vi "Main Controller AM.vi"(8 "Error In":errorcluster) -> (0 "Error Out":errorcluster)   [LabVIEW 2017, in "Main controller.lvlib"]
uses:
  Main controller.lvlib
  Shutter Module/Shutter.lvlib
  Monochromator/Monochromator.lvlib
  UI/UI.lvlib
  DAQ/DAQ.lvlib
  Monochromator/Controls/VISA parameters.ctl
  Serial comms/Serial comms.lvlib
  Monochromator/Controls/Grating.ctl
  Monochromator/Controls/Params.ctl
  DAQ/Controls/Params.ctl
  Scope/Scope.lvlib
  Monochromator/Controls/Type.ctl
  Scope/Controls/TPC.ctl
  Scope/Controls/Models.ctl
  Trigger/Controls/Mode.ctl
  Trigger/Trigger.lvlib
  Trigger/Controls/Params.ctl
  Scope/Controls/Params.ctl
  File IO/File IO.lvlib
  Scope/Controls/Record length.ctl
  Scope/Controls/Acquisition type.ctl
  Trigger channels.ctl
  Colour Wheel/Colour Wheel.lvlib
  Colour Wheel/Controls/Params.ctl
  Scope/Controls/Channel data.ctl
  Scope/Controls/Data.ctl
  Monochromator/Oriel/Controls/Params.ctl
  Monochromator/Oriel/Oriel (old drivers).lvlib
  Monochromator/Custom Oriel drivers/Controls/Params.ctl
  Monochromator/Custom Oriel drivers/Oriel (custom drivers).lvlib
  Monochromator/PTI/Controls/Params.ctl
  Monochromator/PTI/PTI.lvlib
  Monochromator/Controls/GratingValues.ctl
  Events/Events.lvlib
  Events/Controls/Action Refs [enum].ctl
  Test params.ctl
  CTLs/Test indicators.ctl
  Scope/Controls/Channels.ctl
  Processing/Processing.lvlib
  Colour Wheel/Controls/Colours.ctl
  Auto cycle/Controls/Steps.ctl
  Auto cycle/Auto cycle.lvlib
  Auto cycle/Controls/Checks.ctl
  C:/Project Work/icl-optical-software-rewrite/Optical Software Code Simplified/Modules/Monochromator/Cornerstone.dll
  Monochromator/Cornerstone.dll
  Shutter Module/Controls/Params.ctl
  File IO/Controls/Params.ctl
  CTLs/Params.ctl
  CTLs/Test Controls.ctl
  CTLs/Commands [enum].ctl
panel:
  out "Current step":T1
  in  "Commands":T2
  out "Standalone":bool
  out "Config out":T3={"DAQ"={"Data"={"Live"={"t0"=timestamp(0 s since 1904-01-01), "dt"=1.0, "Y"=[]}, "Accumulated"={"t0"=timestamp(0 s since 1904-01-01), "dt"=1.0, "Y"=[]}, "Averaged"={"t0"=timestamp(0 s since 1904-01-01), "dt"=1.0, "Y"=[]}, "data array"=[], "live time array"=[], "Live (decimated)"={"t0"=timestamp(0 s since 1904-01-01), "dt"=1.0, "Y"=[]}}, "Config"={"Input Config"=-1, "Card"=enum."USB-6211", "100% Reflectance Standard (V)"=1.0, "Input Channel"="Dev2/ai0", "Average number of points"=10.0, "Trigger Level (V)"=0.3, "Rate"=250000, "End Time (s)"=1.0}, "Indicators"={"Final number of points"=0.0, "Number of samples"=0.0, "dt"=0.0, "Shots"=1, "Shot counter"=0, "Test counter"=0, "Background level (V)"=0.0, "DAQ task"="", "timestamp of data"=timestamp(0 s since 1904-01-01)}}, "Shutter"={"Open command string"="", "VISA"={"Enable Termination Char (T)"=FALSE, "timeout (ms)"=0, "Resource name"="", "baud rate"=0, "data bits"=0, "parity"=0, "stop bits"=0, "flow control"=0}}, "Monochromator"={"Type"=enum."Oriel", "Wavelength (nm)"=0.0, "Grating, gr/mm"=enum."2400", "Grating mode"=enum."unknown", "Spectrum mode"={"Spectrum mode?"=FALSE, "Start wavelength (nm)"=0.0, "End wavelength (nm)"=0.0, "Wavelength step (nm)"=0.0, "Wavelength array"=[], "array index"=0}, "PTI"={"delay before read (ms)"=0, "Mono 1"={"Enable Termination Char (T)"=FALSE, "timeout (ms)"=0, "Resource name"="", "baud rate"=0, "data bits"=0, "parity"=0, "stop bits"=0, "flow control"=0}, "Mono 2"={"Enable Termination Char (T)"=FALSE, "timeout (ms)"=0, "Resource name"="", "baud rate"=0, "data bits"=0, "parity"=0, "stop bits"=0, "flow control"=0}}, "Oriel (custom)"={"reference"=refnum}, "Oriel (old)"={"configuration file path"=path ""}, "Force wavelength confirmation (PTI)?"=FALSE}, "Test"={"Config"={"Amplification Factor"=0.0, "100% reflectance standard"=0.0, "Calculation Method"=enum."Reflectance", "Option to discard new data?"=FALSE, "Mode"=enum."Spectrum", "Number of averages"=0, "B Test?"=FALSE}, "Indicators"={"DAQ Background Level (V)"=0.0, "A-Test Counter"=0, "B-test counter"=0, "Type"=enum."A-test", "Scope Background Level (Amps)"=2.0, "TAS only?"=FALSE}}, "Scope"={"Config"={"VISA resource"="USB0::0x0699::0x039D::C010764::INSTR", "Model"=enum."DPO 2012B", "Timebase"=0.0004, "Timeout (ms)"=60000, "TAS"={"Vertical Range (10.0 V)"=2.0, "Vertical Offset (0.0 divs)"=0.0, "Bandwidth"=0, "Probe Attenuation (10.0)"=1.0, "Vertical Coupling"=1, "Impedance"=0, "Multiplication factor"=1.0, "Channel"=enum."Channel 1"}, "TPC"={"Vertical Range (10.0 V)"=2.0, "Vertical Offset (0.0 divs)"=0.0, "Bandwidth"=0, "Probe Attenuation (10.0)"=1.0, "Vertical Coupling"=1, "Impedance"=0, "Multiplication factor"=1.0, "Channel"=enum."None"}, "Trigger"={"Mode"=enum."Laser (TAS)", "Source "=enum."Aux", "PIA mode"={"Test LEDs"=FALSE, "LED line"="", "LED off (s)"=0.0, "LED on (s)"=0.0}, "Threshold (V)"=0.8}}, "Indicators"={"Setup"={"Final number of points"=0.0, "Pretrigger points"=0.0, "Number of readouts"=0, "Model"={"Acquisition Type"=4, "Record length (points)"=1000, "Averages on scope"=4, "Average number of points"=10.0}}, "timestamp of data"=timestamp(0 s since 1904-01-01)}, "Data"={"TPC"={"Live data"={"t0"=timestamp(0 s since 1904-01-01), "dt"=1.0, "Y"=[]}, "Averaged data"={"t0"=timestamp(0 s since 1904-01-01), "dt"=1.0, "Y"=[]}, "Accumulated data"={"t0"=timestamp(0 s since 1904-01-01), "dt"=1.0, "Y"=[]}, "Final data"={"t0"=timestamp(0 s since 1904-01-01), "dt"=1.0, "Y"=[]}}, "TAS"={"Live data"={"t0"=timestamp(0 s since 1904-01-01), "dt"=1.0, "Y"=[]}, "Averaged data"={"t0"=timestamp(0 s since 1904-01-01), "dt"=1.0, "Y"=[]}, "Accumulated data"={"t0"=timestamp(0 s since 1904-01-01), "dt"=1.0, "Y"=[]}, "Final data"={"t0"=timestamp(0 s since 1904-01-01), "dt"=1.0, "Y"=[]}}, "Time arrays"={"Time array (decimated)"=[], "waveform"={"t0"=timestamp(0 s since 1904-01-01), "dt"=1.0, "Y"=[]}}}, "Test"={"Config"={"Amplification Factor"=0.0, "100% reflectance standard"=0.0, "Calculation Method"=enum."Reflectance", "Option to discard new data?"=FALSE, "Mode"=enum."Spectrum", "Number of averages"=100}, "Indicators"={"DAQ Background Level (V)"=2.0, "A-Test Counter"=2, "B-test counter"=2, "Type"=enum."A-test", "Scope Background Level (Amps)"=2.0, "TAS only?"=FALSE}, "Stop Measurement"=FALSE, "Stop Measurement 2"=FALSE}}, "Colour wheel"={"Reference"=0, "Wavelength Enum"=enum."435"}, "File IO"={"Output Folder"=path "C:/Users/Abigail/Documents/Imperial Optical software/Optical Software Code Simplified/Output", "Error file"=path "C:/Users/Abigail/Documents/Imperial Optical software/Optical Software Code Simplified/Error Log.txt", "Config file"=path "C:/Users/Abigail/Documents/Imperial Optical software/Optical Software Code Simplified/Config.ini", "File prefix"="", "Waveform read"={"t0"=timestamp(0 s since 1904-01-01), "dt"=1.0, "Y"=[]}}} {"Scope"."Indicators"."Setup"."Model"."Record length (points)" items=["1000"=1, "10,000"=10, "100,000"=100, "1,000,000"=1000, "5,000,000"=5000, "10,000,000"=10000]; "Scope"."Indicators"."Setup"."Model"."Acquisition Type" items=["Sample", "Peak Detect", "Hi Res", "Envelope", "Average"]; "Scope"."Config"."Trigger"."Threshold (V)" format="%#_3f"; "Scope"."Config"."TPC"."Impedance" items=["1M", "75", "50"]; "Scope"."Config"."TPC"."Vertical Coupling" items=["AC", "DC", "Ground"]; "Scope"."Config"."TPC"."Bandwidth" items=["FULL", "250 MHz", "150 MHz", "20 MHz"]; "Scope"."Config"."TAS"."Impedance" items=["1M", "75", "50"]; "Scope"."Config"."TAS"."Vertical Coupling" items=["AC", "DC", "Ground"]; "Scope"."Config"."TAS"."Bandwidth" items=["FULL", "250 MHz", "150 MHz", "20 MHz"]; "Scope"."Config"."Timebase" format="%^#_3e"; "Monochromator"."PTI"."Mono 2"."flow control" items=["None"=0, "XON/XOFF"=1, "RTS/CTS"=2, "DTR/DSR"=4]; "Monochromator"."PTI"."Mono 2"."stop bits" items=["1.0"=10, "1.5"=15, "2.0"=20]; "Monochromator"."PTI"."Mono 2"."parity" items=["None", "Odd", "Even", "Mark", "Space"]; "Monochromator"."PTI"."Mono 1"."flow control" items=["None"=0, "XON/XOFF"=1, "RTS/CTS"=2, "DTR/DSR"=4]; "Monochromator"."PTI"."Mono 1"."stop bits" items=["1.0"=10, "1.5"=15, "2.0"=20]; "Monochromator"."PTI"."Mono 1"."parity" items=["None", "Odd", "Even", "Mark", "Space"]; "Shutter"."VISA"."flow control" items=["None"=0, "XON/XOFF"=1, "RTS/CTS"=2, "DTR/DSR"=4]; "Shutter"."VISA"."stop bits" items=["1.0"=10, "1.5"=15, "2.0"=20]; "Shutter"."VISA"."parity" items=["None", "Odd", "Even", "Mark", "Space"]; "DAQ"."Config"."Input Config" items=["default"=-1, "RSE"=10083, "NRSE"=10078, "Differential"=10106, "Pseudodifferential"=12529]}
  # "#TODO: \"stop[current-test]\""
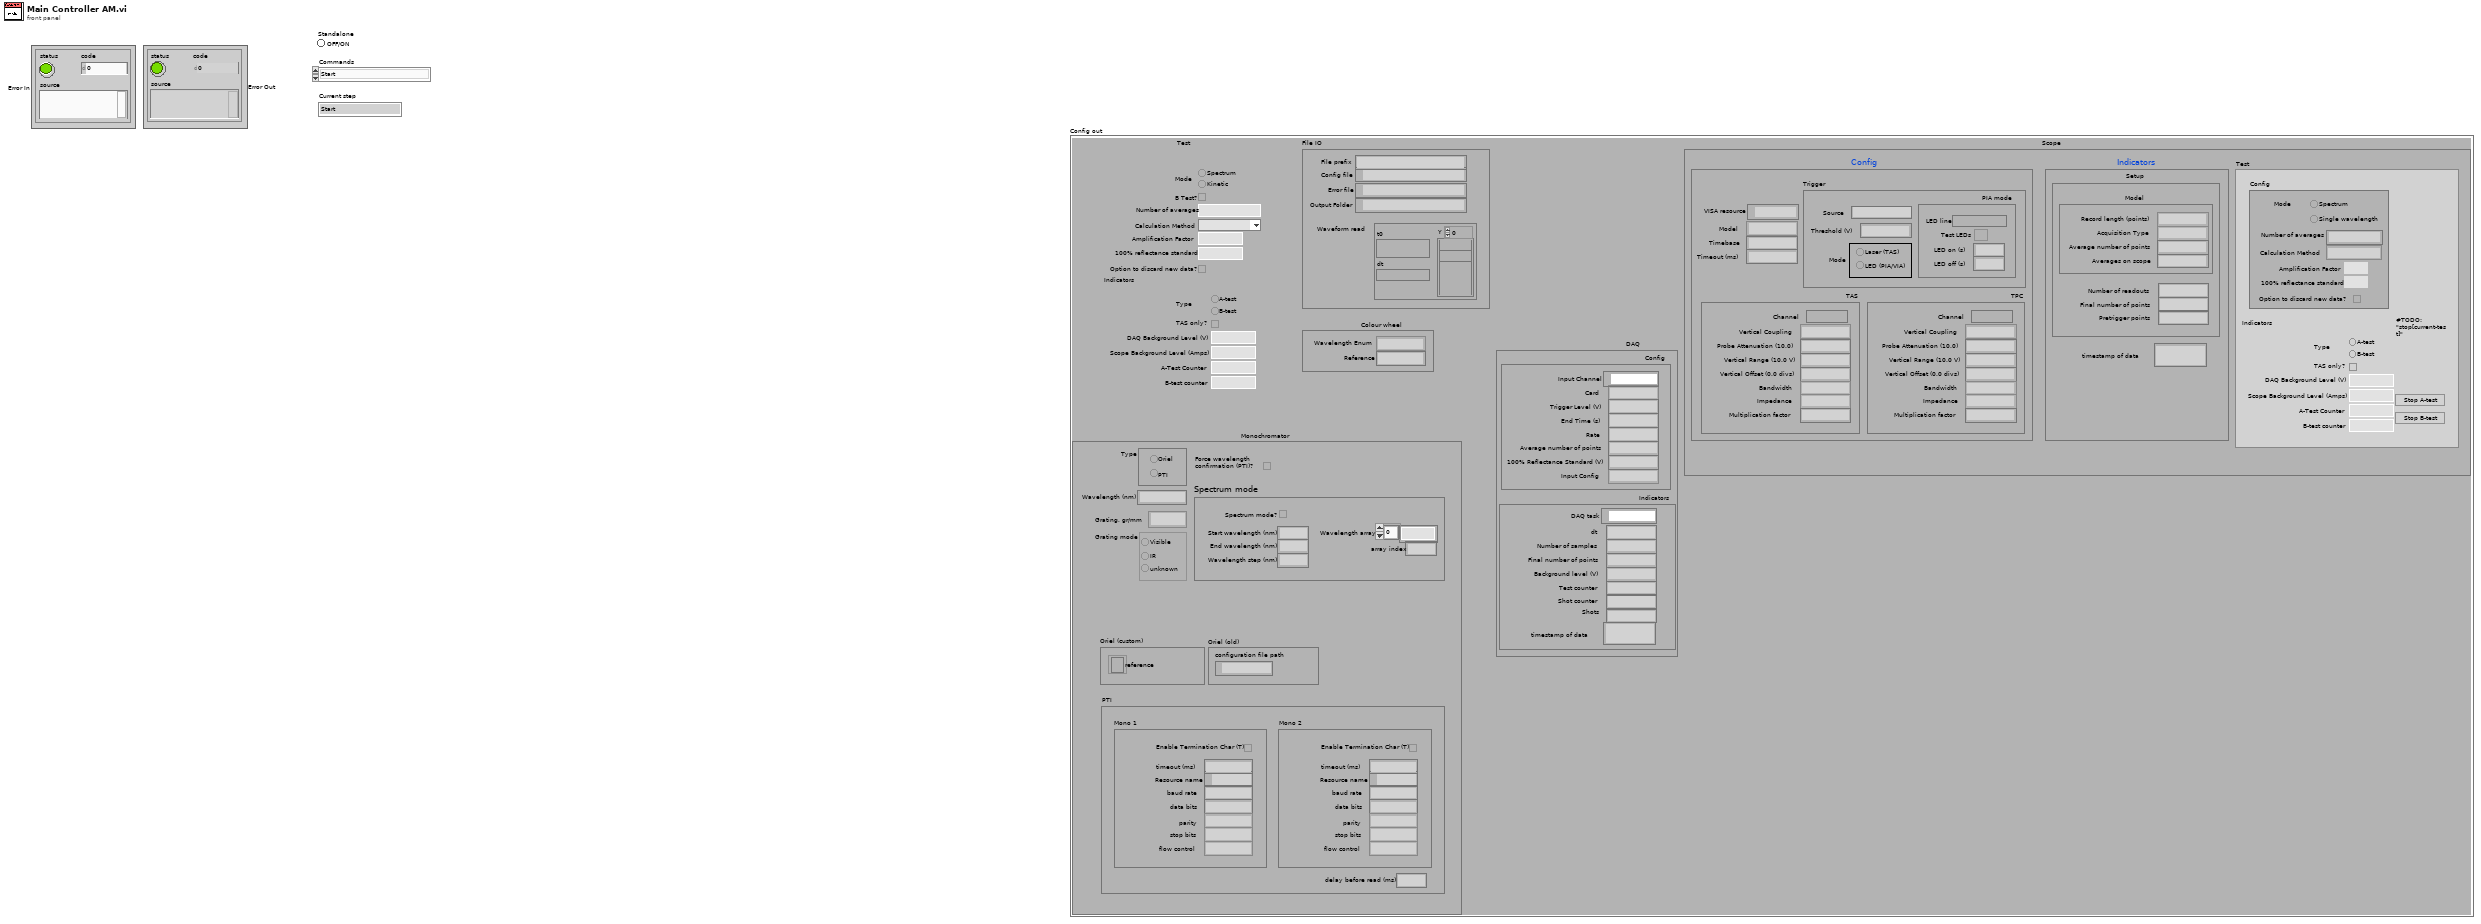
[diagram p1: front panel]
types:
  T1 = typedef "Auto cycle.lvlib/Steps.ctl" = enum16{"Start", "Setup spectrum", "Setup monochromator", "Setup colour wheel", "Move shutter", "Collect data", "Process A or B test", "A-B processing, stitching", "Return shutter"}
  T2 = typedef "Main controller.lvlib/Commands [enum].ctl" = enum16{"Start", "Initialise Devices", "Stop", "Set DAQ data", "Set Scope data", "Set Spectrum Setup", "Spectrum Setup Complete", "Set Monochromator Setup", "Monochromator Setup Complete", "Set Monochromator data", "Set Colour Wheel Setup", "Colour Wheel Setup Complete", "Move Shutter", "Move Shutter Complete", "Collect Data", "DAQ Acquisition Complete", "Scope Acquisition Complete", "Collect Data Complete", "A-B Processing", "A-B Processing Complete", "DAQ-Scope Stitching", "DAQ-Scope Stitching Complete", "Return Shutter", "Return Shutter Complete", "Set colour wheel data", "Set all config data", "Acquire test data", "Accumulate test data", "Average test data", "All Averaging Complete", "DAQ Averaging Complete", "Scope Averaging Complete", "Finalise test data", "All Finalising Complete", "DAQ Finalising Complete", "Scope Finalising Complete", "Process test data"}
  T3 = typedef "Main controller.lvlib/Params.ctl" = cluster{"DAQ":T4, "Shutter":T5, "Monochromator":T7, "Test":T14, "Scope":T17, "Colour wheel":T29, "File IO":T31}
  T4 = typedef "DAQ.lvlib/Params.ctl" = cluster{"Data":cluster{"Live":waveform(dbl), "Accumulated":waveform(dbl), "Averaged":waveform(dbl), "data array":dbl[], "live time array":dbl[], "Live (decimated)":waveform(dbl)}, "Config":cluster{"Input Config":i32, "Card":enum16{"USB-6211", "USB-6251", "USB-6361"}, "100% Reflectance Standard (V)":dbl, "Input Channel":tag, "Average number of points":dbl, "Trigger Level (V)":dbl, "Rate":i32, "End Time (s)":dbl}, "Indicators":cluster{"Final number of points":dbl, "Number of samples":dbl, "dt":dbl, "Shots":i32, "Shot counter":i32, "Test counter":i32, "Background level (V)":dbl, "DAQ task":refnum<k21>, "timestamp of data":timestamp}}
  T5 = typedef "Shutter.lvlib/Params.ctl" = cluster{"Open command string":string, "VISA":T6}
  T6 = typedef "Serial comms.lvlib/VISA parameters.ctl" = cluster{"Enable Termination Char (T)":bool, "timeout (ms)":u32, "Resource name":refnum<visa-resource-name>, "baud rate":u32, "data bits":u16, "parity":u16, "stop bits":u16, "flow control":u16}
  T7 = typedef "Monochromator.lvlib/Params.ctl" = cluster{"Type":T8, "Wavelength (nm)":dbl, "Grating, gr/mm":T9, "Grating mode":T10, "Spectrum mode":cluster{"Spectrum mode?":bool, "Start wavelength (nm)":dbl, "End wavelength (nm)":dbl, "Wavelength step (nm)":dbl, "Wavelength array":dbl[], "array index":u32}, "PTI":T11, "Oriel (custom)":T12, "Oriel (old)":T13, "Force wavelength confirmation (PTI)?":bool}
  T8 = typedef "Monochromator.lvlib/Type.ctl" = enum32{"Oriel", "PTI"}
  T9 = typedef "Monochromator.lvlib/GratingValues.ctl" = enum16{"2400", "1800", "1200", "600", "300", "150"}
  T10 = typedef "Monochromator.lvlib/Grating.ctl" = enum32{"unknown", "Visible", "IR"}
  T11 = typedef "Monochromator.lvlib/PTI.lvlib/Params.ctl" = cluster{"delay before read (ms)":u32, "Mono 1":T6, "Mono 2":T6}
  T12 = typedef "Monochromator.lvlib/Oriel (custom drivers).lvlib/Params.ctl" = cluster{"reference":refnum<k24>}
  T13 = typedef "Monochromator.lvlib/Oriel (old drivers).lvlib/Params.ctl" = cluster{"configuration file path":path}
  T14 = typedef "Test params.ctl" = cluster{"Config":T15, "Indicators":T16}
  T15 = typedef "Main controller.lvlib/Test Controls.ctl" = cluster{"Amplification Factor":dbl, "100% reflectance standard":dbl, "Calculation Method":enum16{"Reflectance", "Transmission", "Kubelka-Munk"}, "Option to discard new data?":bool, "Mode":enum32{"Spectrum", "Kinetic"}, "Number of averages":u32, "B Test?":bool}
  T16 = typedef "Main controller.lvlib/Test indicators.ctl" = cluster{"DAQ Background Level (V)":dbl, "A-Test Counter":i32, "B-test counter":i32, "Type":enum32{"A-test", "B-test"}, "Scope Background Level (Amps)":dbl, "TAS only?":bool}
  T17 = typedef "Scope.lvlib/Params.ctl" = cluster{"Config":cluster{"VISA resource":refnum<visa-resource-name>, "Model":T18, "Timebase":dbl, "Timeout (ms)":u32, "TAS":T19, "TPC":T19, "Trigger":T21}, "Indicators":cluster{"Setup":cluster{"Final number of points":dbl, "Pretrigger points":dbl, "Number of readouts":i32, "Model":cluster{"Acquisition Type":T24, "Record length (points)":T25, "Averages on scope":i32, "Average number of points":dbl}}, "timestamp of data":timestamp}, "Data":T26, "Test":T28}
  T18 = typedef "Scope.lvlib/Models.ctl" = enum16{"DPO 3012", "DPO 2012B", "TDS 3012C"}
  T19 = typedef "Scope.lvlib/TPC.ctl" = cluster{"Vertical Range (10.0 V)":dbl, "Vertical Offset (0.0 divs)":dbl, "Bandwidth":i32, "Probe Attenuation (10.0)":dbl, "Vertical Coupling":u16, "Impedance":u16, "Multiplication factor":dbl, "Channel":T20}
  T20 = typedef "Scope.lvlib/Channels.ctl" = enum16{"Channel 1", "Channel 2", "Channel 3", "Channel 4", "Math", "Reference A", "Reference B", "Reference C", "Reference D", "B1", "B2", "None"}
  T21 = typedef "Scope.lvlib/Trigger.lvlib/Params.ctl" = cluster{"Mode":T22, "Source ":T23, "PIA mode":cluster{"Test LEDs":bool, "LED line":tag, "LED off (s)":dbl, "LED on (s)":dbl}, "Threshold (V)":dbl}
  T22 = typedef "Scope.lvlib/Trigger.lvlib/Mode.ctl" = enum32{"Laser (TAS)", "LED (PIA/VIA)"}
  T23 = typedef "Scope.lvlib/Trigger.lvlib/Trigger channels.ctl" = enum16{"Channel 1", "Channel 2", "Channel 3", "Channel 4", "AC Line", "Aux", "Digital Channel 0", "Digital Channel 1", "Digital Channel 2", "Digital Channel 3", "Digital Channel 4", "Digital Channel 5", "Digital Channel 6", "Digital Channel 7", "Digital Channel 8", "Digital Channel 9", "Digital Channel 10", "Digital Channel 11", "Digital Channel 12", "Digital Channel 13", "Digital Channel 14", "Digital Channel 15", "RF"}
  T24 = typedef "Scope.lvlib/Acquisition type.ctl" = u16
  T25 = typedef "Scope.lvlib/Record length.ctl" = u32
  T26 = typedef "Scope.lvlib/Data.ctl" = cluster{"TPC":T27, "TAS":T27, "Time arrays":cluster{"Time array (decimated)":dbl[], "waveform":waveform(dbl)}}
  T27 = typedef "Scope.lvlib/Channel data.ctl" = cluster{"Live data":waveform(dbl), "Averaged data":waveform(dbl), "Accumulated data":waveform(dbl), "Final data":waveform(dbl)}
  T28 = typedef "Main controller.lvlib/Test params.ctl" = cluster{"Config":cluster{"Amplification Factor":dbl, "100% reflectance standard":dbl, "Calculation Method":enum16{"Reflectance", "Transmission", "Kubelka-Munk"}, "Option to discard new data?":bool, "Mode":enum32{"Spectrum", "Single wavelength"}, "Number of averages":u32}, "Indicators":T16, "Stop Measurement":bool, "Stop Measurement 2":bool}
  T29 = typedef "Colour Wheel.lvlib/Params.ctl" = cluster{"Reference":i32, "Wavelength Enum":T30}
  T30 = typedef "Colour Wheel.lvlib/Colours.ctl" = enum16{"N/A", "435", "590", "665", "715", "850", "1000"}
  T31 = typedef "File IO.lvlib/Params.ctl" = cluster{"Output Folder":path, "Error file":path, "Config file":path, "File prefix":string, "Waveform read":waveform(dbl)}
  T32 = typedef "Auto cycle.lvlib/Checks.ctl" = bool[]
  T33 = enum32{"Bad", "Idle", "Run top level", "Running"}
  T34 = typedef "Events.lvlib/Action Refs [enum].ctl" = enum16{"Init", "Ref", "Kill"}
  T35 = typedef "Events.lvlib/Refs [cluster].ctl" = cluster{"Exit":refnum<user-event>, "Controller":refnum<user-event>, "System Error":refnum<user-event>, "UI":refnum<user-event>, "Example Module":refnum<user-event>, "Shutter":refnum<user-event>, "Monochromator":refnum<user-event>, "DAQ":refnum<user-event>, "Scope":refnum<user-event>, "Auto cycle":refnum<user-event>, "Processing":refnum<user-event>, "File IO":refnum<user-event>, "Colour wheel":refnum<user-event>}
  T36 = typedef "Scope.lvlib/Params.ctl" = cluster{"Config":cluster{"VISA resource":refnum<visa-resource-name>, "Model":T18, "Timebase":dbl, "Timeout (ms)":u32, "TAS":T19, "TPC":T19, "Trigger":T21}, "Indicators":cluster{"Setup":cluster{"Final number of points":dbl, "Pretrigger points":dbl, "Number of readouts":i32, "Model":cluster{"Acquisition Type":T24, "Record length (points)":T25, "Averages on scope":i32, "Average number of points":dbl}}, "timestamp of data":timestamp}, "Data":T26, "Test":cluster{"Config":T15, "Indicators":T16}}
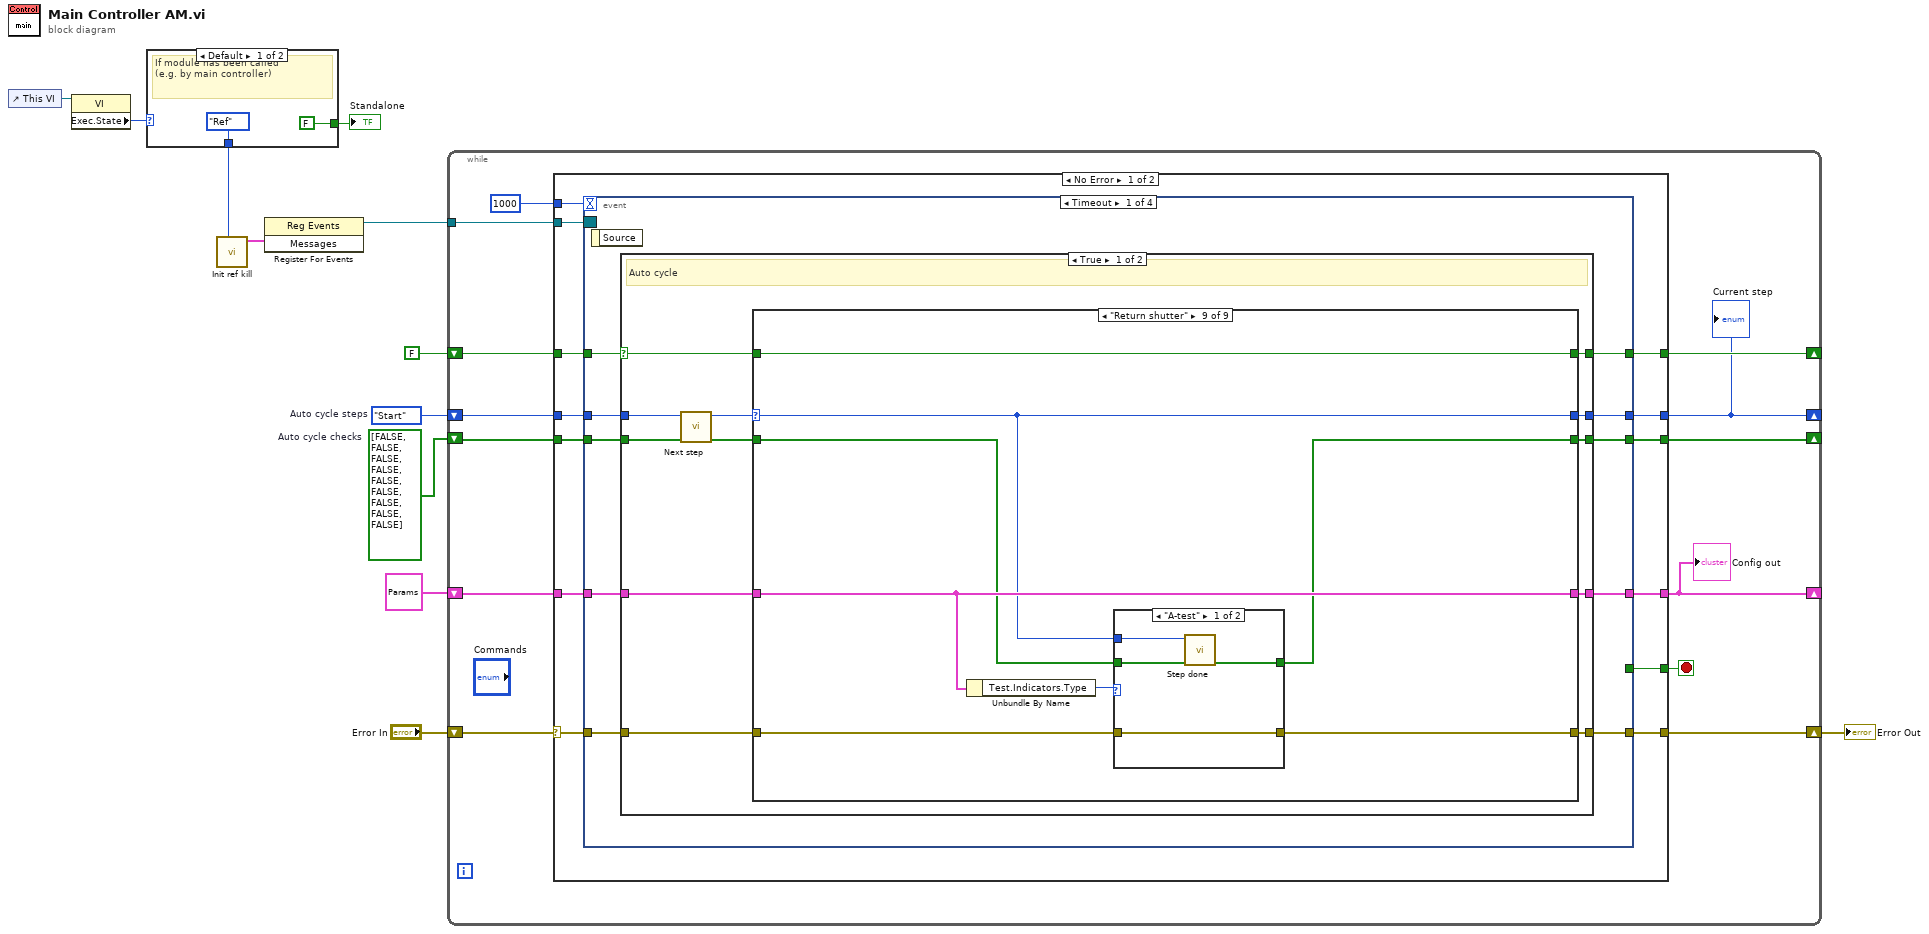
[diagram p0: block diagram]
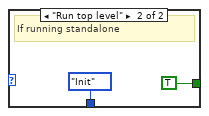
[diagram p2: hidden frame]
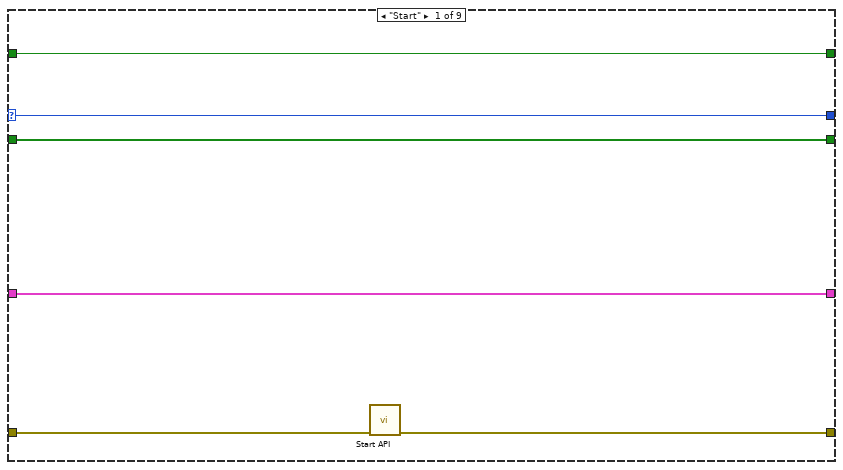
[diagram p3: hidden frame]
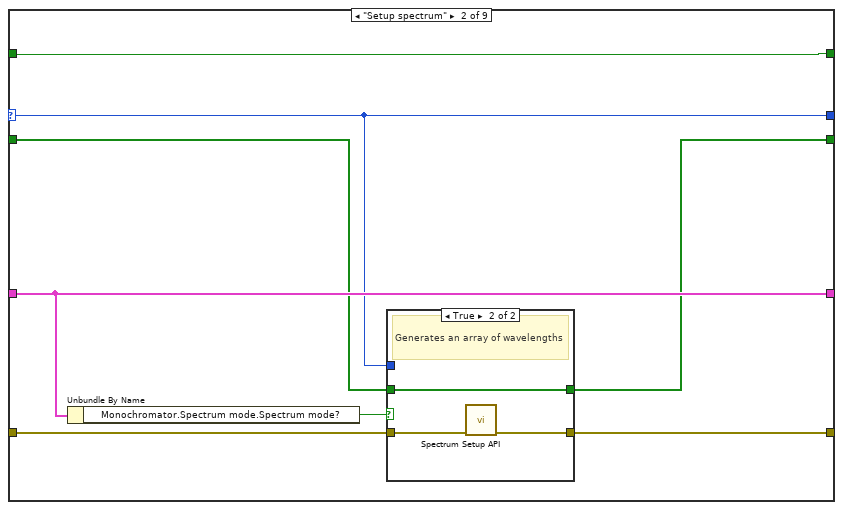
[diagram p4: hidden frame]
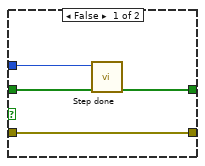
[diagram p5: hidden frame]
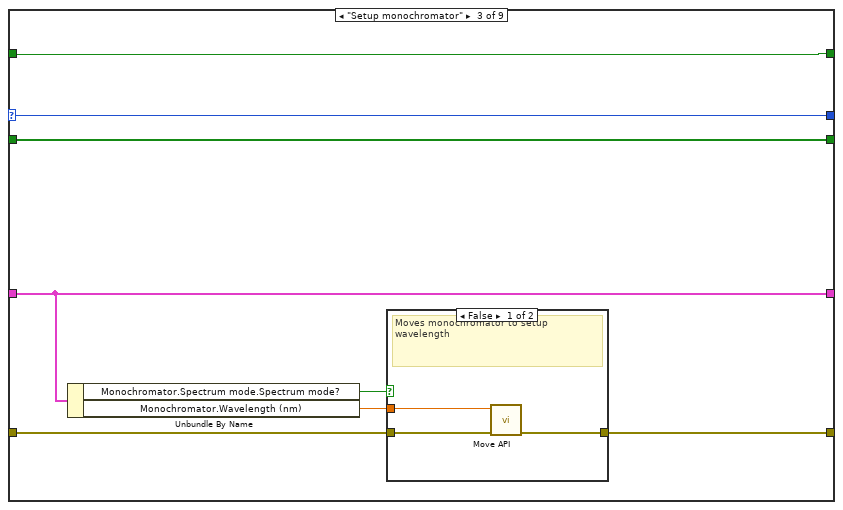
[diagram p6: hidden frame]
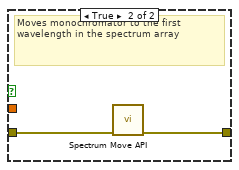
[diagram p7: hidden frame]
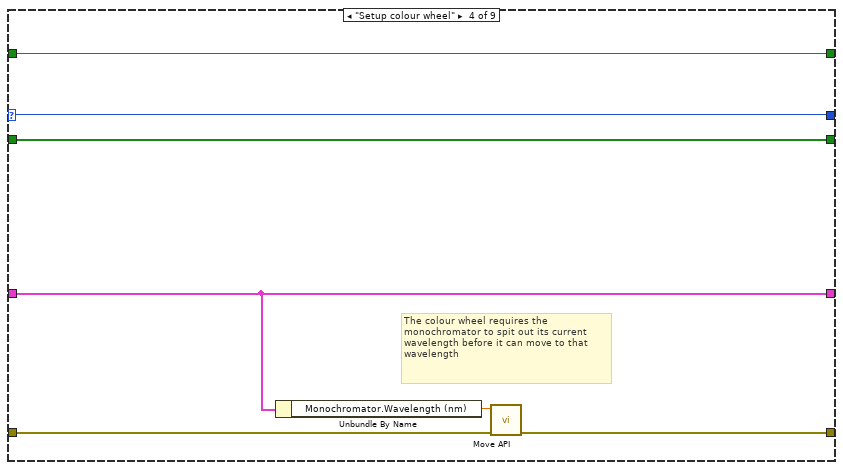
[diagram p8: hidden frame]
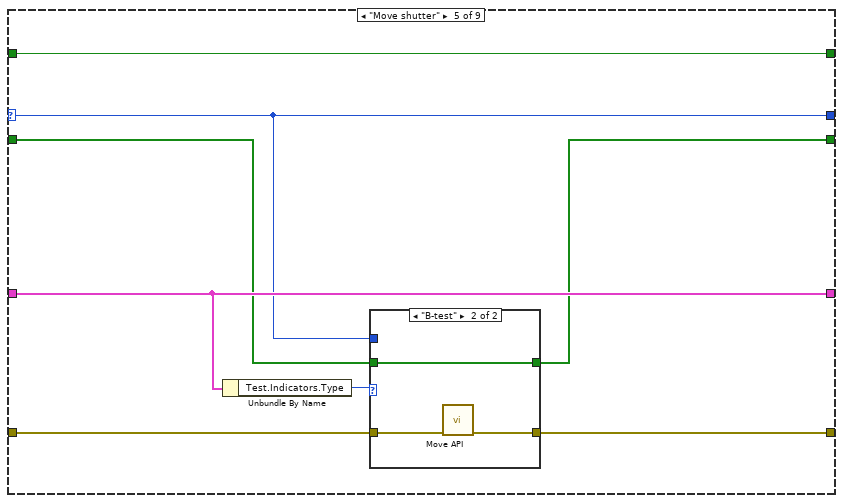
[diagram p9: hidden frame]
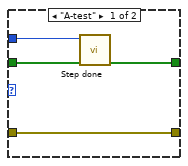
[diagram p10: hidden frame]
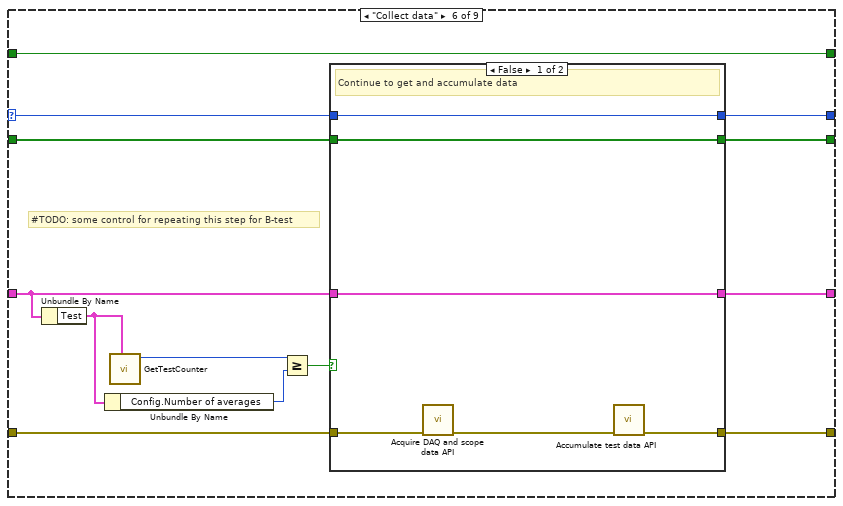
[diagram p11: hidden frame]
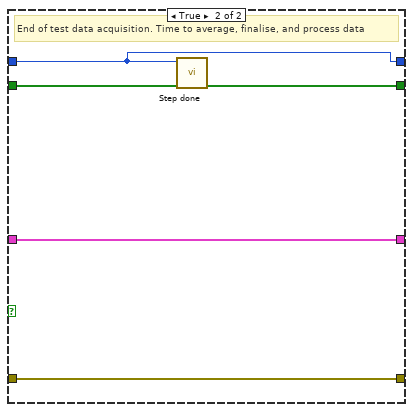
[diagram p12: hidden frame]
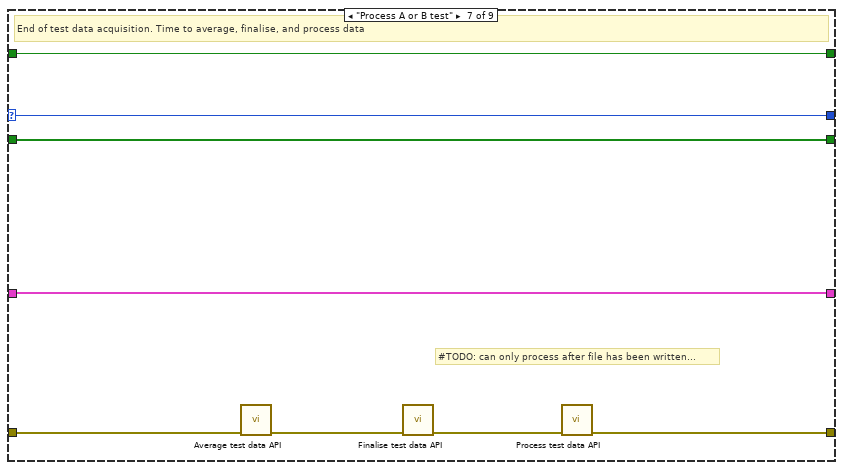
[diagram p13: hidden frame]
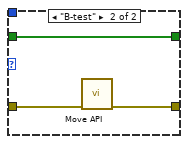
[diagram p15: hidden frame]
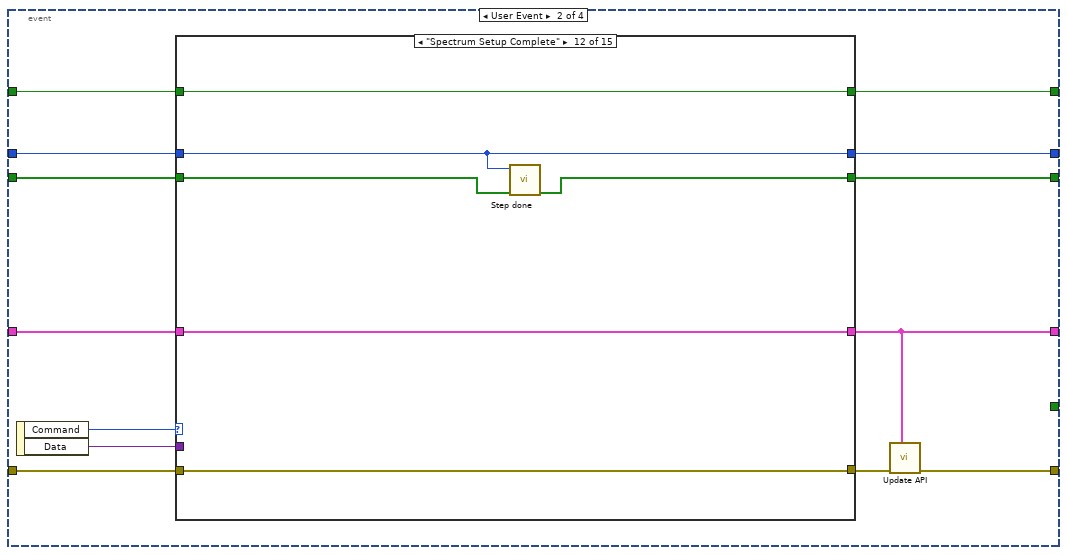
[diagram p17: hidden frame]
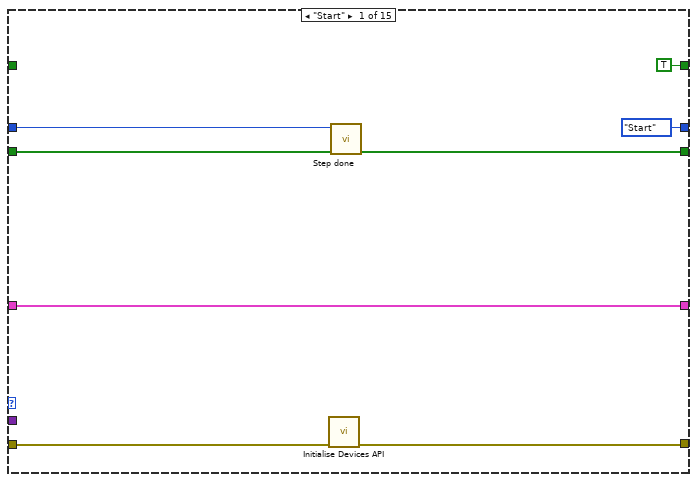
[diagram p18: hidden frame]
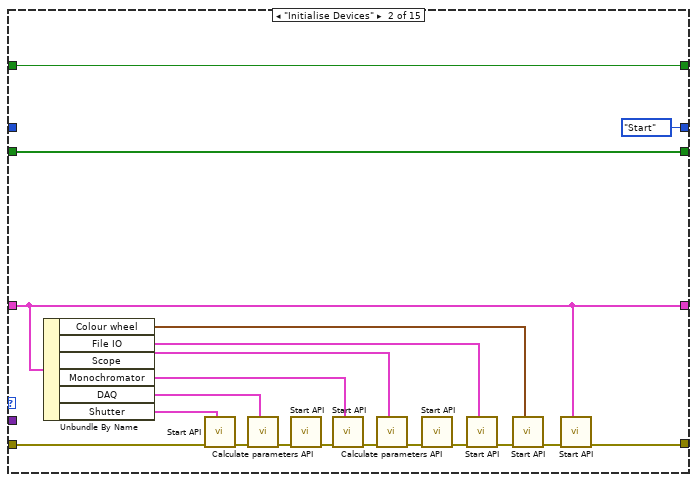
[diagram p19: hidden frame]
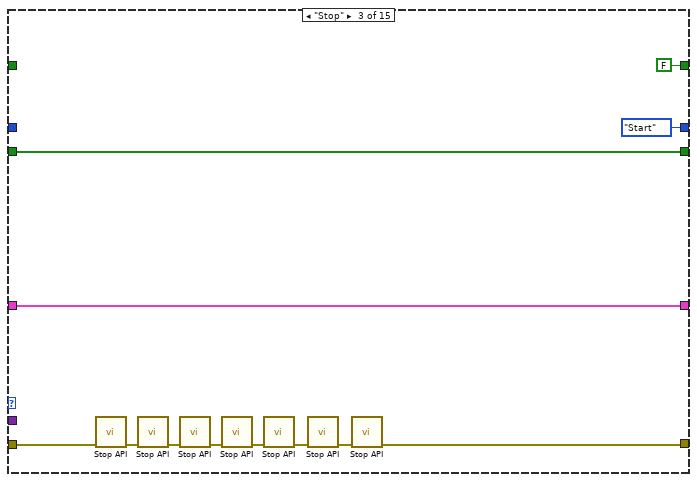
[diagram p20: hidden frame]
diagram:
  w1 = T32 [FALSE, FALSE, FALSE, FALSE, FALSE, FALSE, FALSE, FALSE, FALSE]  # Auto cycle checks
  w2 = Steps."Start"  # Auto cycle steps
  n1 = control-ref of="This VI"() -> (w9:refnum<vi>)
  n2 = property class="VI"(reference=w9) -> ("Exec.State"=w8:T33)  [unwired: 1 in, 2 out]
  n3 = case shown="Default" w8 {
    tunnel: [Action_Refs_[enum]."Ref" ("Action") Action_Refs_[enum]."Init" ("Action")] -> w7
    tunnel: [FALSE TRUE] -> w6
    frame Default {
      # "If module has been called\n(e.g. by main controller)"
    }
    frame "Run top level" {
      # "If running standalone"
    }
  }
  "Standalone" <- w6
  n4 = call "Init ref kill.vi"("Action"=w7) -> ("Messages"=w10:T35)  [unwired: 9 in, 1 out]
  n5 = register-events(w10) -> (reference out=w5:refnum<event-registration>)  [unwired: 2 in, 1 out]
  n6 = while {
    shift-right: [w28] -> w11
    shift-left: "Error In" -> [w23]
    shift-right: [w25] -> _
    shift-left: T3 {"DAQ"={"Data"={"Live"={"t0"=timestamp(0 s since 1904-01-01), "dt"=1.0, "Y"=[]}, "Accumulated"={"t0"=timestamp(0 s since 1904-01-01), "dt"=1.0, "Y"=[]}, "Averaged"={"t0"=timestamp(0 s since 1904-01-01), "dt"=1.0, "Y"=[]}, "data array"=[], "live time array"=[], "Live (decimated)"={"t0"=timestamp(0 s since 1904-01-01), "dt"=1.0, "Y"=[]}}, "Config"={"Input Config"=10106, "Card"=enum."USB-6211", "100% Reflectance Standard (V)"=1.0, "Input Channel"="Dev2/ai0", "Average number of points"=50.0, "Trigger Level (V)"=0.4, "Rate"=250000, "End Time (s)"=1.0}, "Indicators"={"Final number of points"=0.0, "Number of samples"=0.0, "dt"=0.0, "Shots"=1, "Shot counter"=0, "Test counter"=0, "Background level (V)"=0.0, "DAQ task"="", "timestamp of data"=timestamp(0 s since 1904-01-01)}}, "Shutter"={"Open command string"="", "VISA"={"Enable Termination Char (T)"=FALSE, "timeout (ms)"=0, "Resource name"="", "baud rate"=0, "data bits"=0, "parity"=0, "stop bits"=0, "flow control"=0}}, "Monochromator"={"Type"=enum."Oriel", "Wavelength (nm)"=0.0, "Grating, gr/mm"=enum."2400", "Grating mode"=enum."unknown", "Spectrum mode"={"Spectrum mode?"=FALSE, "Start wavelength (nm)"=0.0, "End wavelength (nm)"=0.0, "Wavelength step (nm)"=0.0, "Wavelength array"=[], "array index"=0}, "PTI"={"delay before read (ms)"=0, "Mono 1"={"Enable Termination Char (T)"=FALSE, "timeout (ms)"=0, "Resource name"="", "baud rate"=0, "data bits"=0, "parity"=0, "stop bits"=0, "flow control"=0}, "Mono 2"={"Enable Termination Char (T)"=FALSE, "timeout (ms)"=0, "Resource name"="", "baud rate"=0, "data bits"=0, "parity"=0, "stop bits"=0, "flow control"=0}}, "Oriel (custom)"={"reference"=refnum}, "Oriel (old)"={"configuration file path"=path ""}, "Force wavelength confirmation (PTI)?"=FALSE}, "Test"={"Config"={"Amplification Factor"=0.0, "100% reflectance standard"=0.0, "Calculation Method"=enum."Reflectance", "Option to discard new data?"=FALSE, "Mode"=enum."Spectrum", "Number of averages"=0, "B Test?"=FALSE}, "Indicators"={"DAQ Background Level (V)"=0.0, "A-Test Counter"=0, "B-test counter"=0, "Type"=enum."A-test", "Scope Background Level (Amps)"=2.0, "TAS only?"=FALSE}}, "Scope"={"Config"={"VISA resource"="USB0::0x0699::0x039D::C010764::INSTR", "Model"=enum."DPO 2012B", "Timebase"=0.0004, "Timeout (ms)"=60000, "TAS"={"Vertical Range (10.0 V)"=2.0, "Vertical Offset (0.0 divs)"=0.0, "Bandwidth"=0, "Probe Attenuation (10.0)"=1.0, "Vertical Coupling"=1, "Impedance"=0, "Multiplication factor"=1.0, "Channel"=enum."Channel 1"}, "TPC"={"Vertical Range (10.0 V)"=2.0, "Vertical Offset (0.0 divs)"=0.0, "Bandwidth"=0, "Probe Attenuation (10.0)"=1.0, "Vertical Coupling"=1, "Impedance"=0, "Multiplication factor"=1.0, "Channel"=enum."None"}, "Trigger"={"Mode"=enum."Laser (TAS)", "Source "=enum."Aux", "PIA mode"={"Test LEDs"=FALSE, "LED line"="", "LED off (s)"=0.0, "LED on (s)"=0.0}, "Threshold (V)"=0.8}}, "Indicators"={"Setup"={"Final number of points"=0.0, "Pretrigger points"=0.0, "Number of readouts"=0, "Model"={"Acquisition Type"=4, "Record length (points)"=1000, "Averages on scope"=4, "Average number of points"=10.0}}, "timestamp of data"=timestamp(0 s since 1904-01-01)}, "Data"={"TPC"={"Live data"={"t0"=timestamp(0 s since 1904-01-01), "dt"=1.0, "Y"=[]}, "Averaged data"={"t0"=timestamp(0 s since 1904-01-01), "dt"=1.0, "Y"=[]}, "Accumulated data"={"t0"=timestamp(0 s since 1904-01-01), "dt"=1.0, "Y"=[]}, "Final data"={"t0"=timestamp(0 s since 1904-01-01), "dt"=1.0, "Y"=[]}}, "TAS"={"Live data"={"t0"=timestamp(0 s since 1904-01-01), "dt"=1.0, "Y"=[]}, "Averaged data"={"t0"=timestamp(0 s since 1904-01-01), "dt"=1.0, "Y"=[]}, "Accumulated data"={"t0"=timestamp(0 s since 1904-01-01), "dt"=1.0, "Y"=[]}, "Final data"={"t0"=timestamp(0 s since 1904-01-01), "dt"=1.0, "Y"=[]}}, "Time arrays"={"Time array (decimated)"=[], "waveform"={"t0"=timestamp(0 s since 1904-01-01), "dt"=1.0, "Y"=[]}}}, "Test"={"Config"={"Amplification Factor"=0.0, "100% reflectance standard"=0.0, "Calculation Method"=enum."Reflectance", "Option to discard new data?"=FALSE, "Mode"=enum."Spectrum", "Number of averages"=100}, "Indicators"={"DAQ Background Level (V)"=2.0, "A-Test Counter"=2, "B-test counter"=2, "Type"=enum."A-test", "Scope Background Level (Amps)"=2.0, "TAS only?"=FALSE}, "Stop Measurement"=FALSE, "Stop Measurement 2"=FALSE}}, "Colour wheel"={"Reference"=0, "Wavelength Enum"=enum."435"}, "File IO"={"Output Folder"=path "C:/Users/Abigail/Documents/Imperial Optical software/Optical Software Code Simplified/Output", "Error file"=path "C:/Users/Abigail/Documents/Imperial Optical software/Optical Software Code Simplified/Error Log.txt", "Config file"=path "C:/Users/Abigail/Documents/Imperial Optical software/Optical Software Code Simplified/Config.ini", "File prefix"="", "Waveform read"={"t0"=timestamp(0 s since 1904-01-01), "dt"=1.0, "Y"=[]}}} ("Config") -> [w26]
    tunnel: w5 -> [w24]
    shift-right: [w21] -> _
    shift-left: FALSE -> [w22]
    shift-right: [w20] -> _
    shift-left: w2 -> [w19]
    shift-right: [w17] -> _
    shift-left: w1 -> [w18]
    stop <- w27 stop-if-true
    n7 = case shown="No Error" w23 {
      selector: w23 -> [w36 w399]
      tunnel: 1000 -> [w42 _]
      tunnel: [w41 w398] -> w28
      tunnel: [w40 _] -> w27
      tunnel: w26 -> [w39 w400]
      tunnel: [w38 w400] -> w25
      tunnel: w24 -> [w37 _]
      tunnel: w22 -> [w35 w396]
      tunnel: [w34 w396] -> w21
      tunnel: [w33 w395] -> w20
      tunnel: w19 -> [w32 w395]
      tunnel: w18 -> [w31 w394]
      tunnel: [w30 w394] -> w17
      frame No Error {
        n8 = event shown="[0] Timeout" {
          selector: w37 -> [_ _ _ _]
          dyn-events: _ -> [_ _ _ _]
          timeout: w42 -> [_ _ _ _]
          tunnel: [w51 w184 w351 w393] -> w41
          tunnel: w36 -> [w52 w190 w350 w393]
          tunnel: [_ _ _ TRUE] -> w40
          tunnel: w39 -> [w49 w187 w348 w391]
          tunnel: [w50 w186 w348 w391] -> w38
          tunnel: w35 -> [w48 w181 w347 w390]
          tunnel: [w45 w180 w347 w390] -> w34
          tunnel: [w46 w182 w346 w389] -> w33
          tunnel: w32 -> [w47 w183 w346 w389]
          tunnel: w31 -> [w44 w179 _ _]
          tunnel: [w43 w178 _ _] -> w30
          event Timeout {
            n9 = event-data() -> ()  [unwired: 1 in, 1 out]
            n10 = case shown="True" w48 {
              selector: w48 -> [w64 w174]
              tunnel: w52 -> [w60 w176]
              tunnel: [w59 w176] -> w51
              tunnel: [w62 w177] -> w50
              tunnel: w49 -> [w61 w177]
              tunnel: w47 -> [w56 w175]
              tunnel: [w58 w175] -> w46
              tunnel: [w63 w174] -> w45
              tunnel: w44 -> [w53 w173]
              tunnel: [w57 w173] -> w43
              frame True {
                # "Auto cycle"
                n11 = call "Next step.vi"("Auto cycle checks in"=w53, "Auto cycle step in"=w56) -> ("Auto cycle checks out"=w54:T32, "Auto cycle step out"=w55:T1)  [unwired: 8 in]
                n12 = case shown="\"Return shutter\"" w55 {
                  selector: w55 -> [w65 w73 w86 w99 w107 w125 w145 w153 w159]
                  tunnel: w64 -> [w70 w74 w88 w101 w113 w133 w152 w157 w165]
                  tunnel: [w70 w74 w88 w101 w113 w133 w152 w157 w165] -> w63
                  tunnel: [w69 w78 w93 w105 w110 w127 w151 w156 w162] -> w62
                  tunnel: w61 -> [w69 w78 w93 w105 w110 w121 w151 w156 w162]
                  tunnel: w60 -> [w68 w77 w92 w104 w112 w129 w147 w155 w164]
                  tunnel: [w67 w76 w91 w103 w111 w128 w146 w155 w163] -> w59
                  tunnel: [w65 w73 w86 w99 w107 w122 w145 w153 w159] -> w58
                  tunnel: w54 -> [w66 w72 w87 w100 w108 w124 w150 w154 w160]
                  tunnel: [w66 w71 w87 w100 w106 w123 w150 w154 w158] -> w57
                  frame "Start" {
                    n13 = call "Start API.vi"("Error In"=w68) -> ("Error Out"=w67:errorcluster)  [unwired: 10 in]
                  }
                  frame "Setup spectrum" {
                    n14 = Unbundle By Name(w78) -> ("Monochromator.Spectrum mode.Spectrum mode?"=w75:bool)
                    n15 = case shown="True" w75 {
                      tunnel: [w82 w84] -> w76
                      tunnel: w77 -> [w82 w85]
                      tunnel: w73 -> [w81 _]
                      tunnel: w72 -> [w80 w83]
                      tunnel: [w79 w83] -> w71
                      frame False {
                        n16 = call "Step done.vi"("Auto cycle checks in"=w80, "Auto cycle step"=w81) -> ("Auto cycle checks out"=w79:T32)  [unwired: 9 in]
                      }
                      frame True {
                        # "Generates an array of wavelengths"
                        n17 = call "Spectrum Setup API.vi"("Error In"=w85) -> ("Error Out"=w84:errorcluster)  [unwired: 10 in]
                      }
                    }
                  }
                  frame "Setup monochromator" {
                    n18 = Unbundle By Name(w93) -> ("Monochromator.Spectrum mode.Spectrum mode?"=w90:bool, "Monochromator.Wavelength (nm)"=w89:dbl)
                    n19 = case shown="False" w90 {
                      tunnel: [w94 w98] -> w91
                      tunnel: w92 -> [w95 w97]
                      tunnel: w89 -> [w96 _]
                      frame False {
                        # "Moves monochromator to setup wavelength"
                        n20 = call "Move API.vi"("Error In"=w95, "wavelength"=w96) -> ("Error Out"=w94:errorcluster)  [unwired: 9 in]
                      }
                      frame True {
                        # "Moves monochromator to the first wavelength in the spectrum array"
                        n21 = call "Spectrum Move API.vi"("Error In"=w97) -> ("Error Out"=w98:errorcluster)  [unwired: 10 in]
                      }
                    }
                  }
                  frame "Setup colour wheel" {
                    # "The colour wheel requires the monochromator to spit out its current wavelength before it can move to that wavelength"
                    n22 = Unbundle By Name(w105) -> ("Monochromator.Wavelength (nm)"=w102:dbl)
                    n23 = call "Move API.vi"("Error In"=w104, "Wavelength enum"=w102) -> ("Error Out"=w103:errorcluster)  [unwired: 9 in]
                  }
                  frame "Move shutter" {
                    n24 = Unbundle By Name(w110) -> ("Test.Indicators.Type"=w109:enum32{"A-test", "B-test"})
                    n25 = case shown="\"B-test\"" w109 {
                      tunnel: w112 -> [w117 w120]
                      tunnel: [w117 w119] -> w111
                      tunnel: w107 -> [w116 _]
                      tunnel: w108 -> [w115 w118]
                      tunnel: [w114 w118] -> w106
                      frame "A-test" {
                        n26 = call "Step done.vi"("Auto cycle checks in"=w115, "Auto cycle step"=w116) -> ("Auto cycle checks out"=w114:T32)  [unwired: 9 in]
                      }
                      frame "B-test" {
                        n27 = call "Move API.vi"("Error In"=w120) -> ("Error Out"=w119:errorcluster)  [unwired: 10 in]
                      }
                    }
                  }
                  frame "Collect data" {
                    # "#TODO: some control for repeating this step for B-test"
                    n28 = Unbundle By Name(w121) -> ("Test"=w126:T14)
                    n29 = Unbundle By Name(w126) -> ("Config.Number of averages"=w131:u32)
                    n30 = call "GetTestCounter.vi"("Test"=w126) -> ("Current test counter"=w132:i32)  [unwired: 10 in]
                    n31 = Greater Or Equal?(x=w132, y=w131) -> (x >= y?=w130:bool)
                    n32 = case shown="False" w130 {
                      tunnel: [w136 w144] -> w127
                      tunnel: w121 -> [w136 w144]
                      tunnel: [w137 w140] -> w128
                      tunnel: w129 -> [w138 w140]
                      tunnel: w124 -> [w134 w143]
                      tunnel: w125 -> [w135 w141]
                      tunnel: [w134 w142] -> w123
                      tunnel: [w135 w141] -> w122
                      frame False {
                        # "Continue to get and accumulate data"
                        n33 = call "Acquire DAQ and scope data API.vi"("Error In"=w138) -> ("Error Out"=w139:errorcluster)  [unwired: 10 in]
                        n34 = call "Accumulate test data API.vi"("Error In"=w139) -> ("Error Out"=w137:errorcluster)  [unwired: 10 in]
                      }
                      frame True {
                        # "End of test data acquisition. Time to average, finalise, and process data"
                        n35 = call "Step done.vi"("Auto cycle checks in"=w143, "Auto cycle step"=w141) -> ("Auto cycle checks out"=w142:T32)  [unwired: 9 in]
                      }
                    }
                  }
                  frame "Process A or B test" {
                    # "#TODO: can only process after file has been written..."
                    # "End of test data acquisition. Time to average, finalise, and process data"
                    n36 = call "Average test data API.vi"("Error In"=w147) -> ("Error Out"=w148:errorcluster)  [unwired: 10 in]
                    n37 = call "Finalise test data API.vi"("Error In"=w148) -> ("Error Out"=w149:errorcluster)  [unwired: 10 in]
                    n38 = call "Process test data API.vi"("Error In"=w149) -> ("Error Out"=w146:errorcluster)  [unwired: 10 in]
                  }
                  frame "A-B processing, stitching" {
                    # "#TODO: this has not been written yet. Good luck..."
                  }
                  frame "Return shutter" {
                    n39 = Unbundle By Name(w162) -> ("Test.Indicators.Type"=w161:enum32{"A-test", "B-test"})
                    n40 = case shown="\"A-test\"" w161 {
                      tunnel: w164 -> [w169 w172]
                      tunnel: [w169 w171] -> w163
                      tunnel: w159 -> [w168 _]
                      tunnel: w160 -> [w167 w170]
                      tunnel: [w166 w170] -> w158
                      frame "A-test" {
                        n41 = call "Step done.vi"("Auto cycle checks in"=w167, "Auto cycle step"=w168) -> ("Auto cycle checks out"=w166:T32)  [unwired: 9 in]
                      }
                      frame "B-test" {
                        n42 = call "Move API.vi"("Error In"=w172) -> ("Error Out"=w171:errorcluster)  [unwired: 10 in]
                      }
                    }
                  }
                }
              }
              frame False {
              }
            }
          }
          event User Event {
            n43 = event-data() -> ("Command"=w189:T2, "Data"=w188:variant)  [unwired: 1 in]
            n44 = case shown="\"Spectrum Setup Complete\"" w189 {
              tunnel: w190 -> [w195 w201 w228 w241 w252 w259 w272 w281 w292 w298 w315 w321 w332 w340 w345]
              tunnel: [w194 w203 w221 w235 w247 w260 w269 w278 w290 w297 w308 w321 w325 w338 w345] -> w185
              tunnel: w188 -> [_ _ _ w240 w251 _ _ _ _ _ w314 _ w331 w339 _]
              tunnel: w187 -> [w196 w202 w227 w237 w249 w258 w273 w282 w293 w304 w312 w320 w329 w336 w344]
              tunnel: [w196 w202 w227 w234 w246 w258 w273 w282 w293 w304 w311 w320 w328 w337 w344] -> w186
              tunnel: w183 -> [w193 _ _ w233 w244 w255 w267 w276 w285 w296 w307 w316 w324 w335 w343]
              tunnel: [Steps."Start" ("Auto cycle steps") Steps."Start" ("Auto cycle steps") Steps."Start" ("Auto cycle steps") w233 w244 w255 w267 w276 w285 w296 w307 w316 w324 w335 w343] -> w182
              tunnel: w181 -> [_ w218 _ w232 w243 w254 w266 w275 w284 w295 w306 w319 w323 w334 w342]
              tunnel: [TRUE w218 FALSE w232 w243 w254 w266 w275 w284 w295 w306 w319 w323 w334 w342] -> w180
              tunnel: w179 -> [w192 w199 w220 w231 w242 w253 w265 w274 w283 w294 w305 w318 w322 w333 w341]
              tunnel: [w191 w199 w220 w231 w242 w253 w265 w274 w283 w294 w305 w317 w322 w333 w341] -> w178
              frame "Start" {
                n45 = call "Initialise Devices API.vi"("Error In"=w195) -> ("Error Out"=w194:errorcluster)  [unwired: 10 in]
                n46 = call "Step done.vi"("Auto cycle checks in"=w192, "Auto cycle step"=w193) -> ("Auto cycle checks out"=w191:T32)  [unwired: 9 in]
              }
              frame "Initialise Devices" {
                n47 = Unbundle By Name(w202) -> ("Colour wheel"=w211:T29, "File IO"=w208:T31, "Scope"=w215:T17, "Monochromator"=w206:T7, "DAQ"=w214:T4, "Shutter"=w205:T5)
                n48 = call "Start API.vi"("Shutter"=w205, "Error In"=w201) -> ("Error Out"=w212:errorcluster)  [unwired: 9 in]
                n49 = call "Calculate parameters API.vi"("DAQ"=w214, "Error In"=w212) -> ("Error Out"=w213:errorcluster)  [unwired: 9 in]
                n50 = call "Start API.vi"("Error In"=w213) -> ("Error Out"=w204:errorcluster)  [unwired: 10 in]
                n51 = call "Start API.vi"("Monochromator"=w206, "Error In"=w204) -> ("Error Out"=w207:errorcluster)  [unwired: 9 in]
                n52 = call "Calculate parameters API.vi"("Scope"=w215, "Error In"=w207) -> ("Error Out"=w216:errorcluster)  [unwired: 9 in]
                n53 = call "Start API.vi"("Error In"=w216) -> ("Error Out"=w217:errorcluster)  [unwired: 10 in]
                n54 = call "Start API.vi"("File IO parameters"=w208, "Error In"=w217) -> ("Error Out"=w209:errorcluster)  [unwired: 9 in]
                n55 = call "Start API.vi"("Colour wheel"=w211, "Error In"=w209) -> ("Error Out"=w210:errorcluster)  [unwired: 9 in]
                n56 = call "Start API.vi"("Config"=w202, "Error In"=w210) -> ("Error Out"=w203:errorcluster)  [unwired: 9 in]
              }
              frame "Stop" {
                n57 = call "Stop API.vi"("Error In"=w228) -> ("Error Out"=w230:errorcluster)  [unwired: 10 in]
                n58 = call "Stop API.vi"("Error In"=w230) -> ("Error Out"=w229:errorcluster)  [unwired: 10 in]
                n59 = call "Stop API.vi"("Error In"=w229) -> ("Error Out"=w226:errorcluster)  [unwired: 10 in]
                n60 = call "Stop API.vi"("Error In"=w226) -> ("Error Out"=w225:errorcluster)  [unwired: 10 in]
                n61 = call "Stop API.vi"("Error In"=w225) -> ("Error Out"=w224:errorcluster)  [unwired: 10 in]
                n62 = call "Stop API.vi"("Error In"=w224) -> ("Error Out"=w223:errorcluster)  [unwired: 10 in]
                n63 = call "Stop API.vi"("Error In"=w223) -> ("Error Out"=w221:errorcluster)  [unwired: 10 in]
              }
              frame "Set DAQ data" {
                n64 = Variant To Data(error in=w241, type=T4 {"Data"={"Live"={"t0"=timestamp(0 s since 1904-01-01), "dt"=1.0, "Y"=[]}, "Accumulated"={"t0"=timestamp(0 s since 1904-01-01), "dt"=1.0, "Y"=[]}, "Averaged"={"t0"=timestamp(0 s since 1904-01-01), "dt"=1.0, "Y"=[]}, "data array"=[], "live time array"=[], "Live (decimated)"={"t0"=timestamp(0 s since 1904-01-01), "dt"=1.0, "Y"=[]}}, "Config"={"Input Config"=0, "Card"=enum."USB-6211", "100% Reflectance Standard (V)"=0.0, "Input Channel"="", "Average number of points"=0.0, "Trigger Level (V)"=0.0, "Rate"=0, "End Time (s)"=0.0}, "Indicators"={"Final number of points"=0.0, "Number of samples"=0.0, "dt"=0.0, "Shots"=10, "Shot counter"=10, "Test counter"=10, "Background level (V)"=0.0, "DAQ task"="", "timestamp of data"=timestamp(0 s since 1904-01-01)}} ("DAQ"), Variant=w240) -> (data=w238:T4, error out=w235:errorcluster)
                n65 = Bundle By Name(cluster=w237, "DAQ"=w238) -> (w234:T3)
                n66 = One Button Dialog(message="DAQ config updated") -> ()  [unwired: 1 in, 1 out]
              }
              frame "Set Scope data" {
                # "Updates the main controller's scope config"
                n67 = Variant To Data(error in=w252, type=T36 {"Config"={"VISA resource"="COM1", "Model"=enum."DPO 2012B", "Timebase"=0.2, "Timeout (ms)"=0, "TAS"={"Vertical Range (10.0 V)"=0.0, "Vertical Offset (0.0 divs)"=0.0, "Bandwidth"=0, "Probe Attenuation (10.0)"=0.0, "Vertical Coupling"=1, "Impedance"=2, "Multiplication factor"=1.0, "Channel"=enum."Channel 1"}, "TPC"={"Vertical Range (10.0 V)"=0.2, "Vertical Offset (0.0 divs)"=0.0, "Bandwidth"=0, "Probe Attenuation (10.0)"=0.0, "Vertical Coupling"=1, "Impedance"=1, "Multiplication factor"=2.0, "Channel"=enum."B1"}, "Trigger"={"Mode"=enum."Laser (TAS)", "Source "=enum."Channel 1", "PIA mode"={"Test LEDs"=FALSE, "LED line"="", "LED off (s)"=0.0, "LED on (s)"=0.0}, "Threshold (V)"=10000.0}}, "Indicators"={"Setup"={"Final number of points"=10000.0, "Pretrigger points"=1000.0, "Number of readouts"=0, "Model"={"Acquisition Type"=2, "Record length (points)"=10, "Averages on scope"=1, "Average number of points"=10000.0}}, "timestamp of data"=timestamp(0 s since 1904-01-01)}, "Data"={"TPC"={"Live data"={"t0"=timestamp(0 s since 1904-01-01), "dt"=1.0, "Y"=[]}, "Averaged data"={"t0"=timestamp(0 s since 1904-01-01), "dt"=1.0, "Y"=[]}, "Accumulated data"={"t0"=timestamp(0 s since 1904-01-01), "dt"=1.0, "Y"=[]}, "Final data"={"t0"=timestamp(0 s since 1904-01-01), "dt"=1.0, "Y"=[]}}, "TAS"={"Live data"={"t0"=timestamp(0 s since 1904-01-01), "dt"=1.0, "Y"=[]}, "Averaged data"={"t0"=timestamp(0 s since 1904-01-01), "dt"=1.0, "Y"=[]}, "Accumulated data"={"t0"=timestamp(0 s since 1904-01-01), "dt"=1.0, "Y"=[]}, "Final data"={"t0"=timestamp(0 s since 1904-01-01), "dt"=1.0, "Y"=[]}}, "Time arrays"={"Time array (decimated)"=[], "waveform"={"t0"=timestamp(0 s since 1904-01-01), "dt"=1.0, "Y"=[]}}}, "Test"={"Config"={"Amplification Factor"=2.0, "100% reflectance standard"=2.0, "Calculation Method"=enum."Kubelka-Munk", "Option to discard new data?"=FALSE, "Mode"=enum."Spectrum", "Number of averages"=0, "B Test?"=FALSE}, "Indicators"={"DAQ Background Level (V)"=2.0, "A-Test Counter"=2, "B-test counter"=2, "Type"=enum."A-test", "Scope Background Level (Amps)"=2.0, "TAS only?"=FALSE}}} ("Scope"), Variant=w251) -> (data=w250:T36, error out=w247:errorcluster)
                n68 = Bundle By Name(cluster=w249, "Scope"=w250) -> (w246:T3)
                n69 = One Button Dialog(message="Scope config updated") -> ()  [unwired: 1 in, 1 out]
              }
              frame "Acquire test data" {
                n70 = Unbundle By Name(w258) -> ("Scope"=w257:T17)
                n71 = Unbundle By Name(w257) -> ("Indicators.Setup.Model.Averages on scope"=w256:i32)
                n72 = call "Start acquisition API.vi"("Error In"=w259) -> ("Error Out"=w263:errorcluster)  [unwired: 10 in]
                n73 = call "Get test data API.vi"("Error In"=w263) -> ("Error Out"=w262:errorcluster)  [unwired: 10 in]
                n74 = call "Get test data API.vi"("Error In"=w259, "Shots"=w256) -> ("Error Out"=w261:errorcluster)  [unwired: 9 in]
                n75 = One Button Dialog(message="Acquiring DAQ/scope data") -> ()  [unwired: 1 in, 1 out]
                n76 = Merge Errors(w262, w261) -> (w260:errorcluster)
              }
              frame "Accumulate test data" {
                n77 = call "Accumulate data API.vi"("Error In"=w272) -> ("Error Out"=w271:errorcluster)  [unwired: 10 in]
                n78 = call "Accumulate data API.vi"("Error In"=w272) -> ("Error Out"=w270:errorcluster)  [unwired: 10 in]
                n79 = Merge Errors(w271, w270) -> (w269:errorcluster)
                n80 = One Button Dialog(message="Accumulating DAQ/scope data") -> ()  [unwired: 1 in, 1 out]
              }
              frame "Average test data" {
                n81 = call "Average data API.vi"("Error In"=w281) -> ("Error Out"=w280:errorcluster)  [unwired: 10 in]
                n82 = call "Average data API.vi"("Error In"=w281) -> ("Error Out"=w279:errorcluster)  [unwired: 10 in]
                n83 = Merge Errors(w280, w279) -> (w278:errorcluster)
                n84 = One Button Dialog(message="Averaging DAQ/scope data") -> ()  [unwired: 1 in, 1 out]
              }
              frame "Finalise test data" {
                n85 = call "Background voltage API.vi"("Error In"=w292) -> ("Error Out"=w291:errorcluster)  [unwired: 10 in]
                n86 = call "Calculate background voltage API.vi"("Error In"=w292) -> ("Error Out"=w288:errorcluster)  [unwired: 10 in]
                n87 = call "Add background voltage API.vi"("Error In"=w288) -> ("Error Out"=w287:errorcluster)  [unwired: 10 in]
                n88 = call "Scale TPC API.vi"("Error In"=w287) -> ("Error Out"=w286:errorcluster)  [unwired: 10 in]
                n89 = Merge Errors(w291, w286) -> (w290:errorcluster)
                n90 = One Button Dialog(message="Finalising DAQ/scope data") -> ()  [unwired: 1 in, 1 out]
              }
              frame "Process test data" {
                w301 = "TAS (final)" ("DAQ average file")
                w302 = "DAQ (averaged)" ("DAQ average file")
                # "Read the scope text file and process it (creates a new \"processed\" file)"
                # "Read the DAQ text file and process it (creates a new \"processed\" file)"
                n91 = call "Read waveform API.vi"("Error In"=w298, "Waveform name"=w302) -> ("Error Out"=w303:errorcluster)  [unwired: 9 in]
                n92 = call "Send waveform API.vi"("Error In"=w303, "Waveform name"=w302) -> ("Error Out"=w300:errorcluster)  [unwired: 9 in]
                n93 = call "Read waveform API.vi"("Error In"=w300, "Waveform name"=w301) -> ("Error Out"=w299:errorcluster)  [unwired: 9 in]
                n94 = call "Send waveform API.vi"("Error In"=w299, "Waveform name"=w301) -> ("Error Out"=w297:errorcluster)  [unwired: 9 in]
              }
              frame "Set Monochromator data" {
                n95 = Variant To Data(error in=w315, type=T7 {"Type"=enum."PTI", "Wavelength (nm)"=600.0, "Grating, gr/mm"=enum."1200", "Grating mode"=enum."unknown", "Spectrum mode"={"Spectrum mode?"=FALSE, "Start wavelength (nm)"=0.0, "End wavelength (nm)"=0.0, "Wavelength step (nm)"=0.0, "Wavelength array"=[], "array index"=0}, "PTI"={"delay before read (ms)"=50, "Mono 1"={"Enable Termination Char (T)"=FALSE, "timeout (ms)"=1000, "Resource name"="COM1", "baud rate"=9600, "data bits"=8, "parity"=0, "stop bits"=10, "flow control"=0}, "Mono 2"={"Enable Termination Char (T)"=FALSE, "timeout (ms)"=1000, "Resource name"="COM1", "baud rate"=9600, "data bits"=8, "parity"=0, "stop bits"=10, "flow control"=0}}, "Oriel (custom)"={"reference"=refnum}, "Oriel (old)"={"configuration file path"=path ""}, "Force wavelength confirmation (PTI)?"=FALSE} ("Monochromator"), Variant=w314) -> (data=w313:T7, error out=w308:errorcluster)
                n96 = Bundle By Name(cluster=w312, "Monochromator"=w313) -> (w311:T3)
                n97 = One Button Dialog(message="Got monochromator data") -> ()  [unwired: 1 in, 1 out]
              }
              frame "Spectrum Setup Complete" {
                n98 = call "Step done.vi"("Auto cycle checks in"=w318, "Auto cycle step"=w316) -> ("Auto cycle checks out"=w317:T32)  [unwired: 9 in]
              }
              frame "Set colour wheel data" {
                n99 = Variant To Data(error in=w332, type=T29 {"Reference"=600, "Wavelength Enum"=enum."435"} ("Colour wheel"), Variant=w331) -> (data=w330:T29, error out=w325:errorcluster)
                n100 = Bundle By Name(cluster=w329, "Colour wheel"=w330) -> (w328:T3)
                n101 = One Button Dialog(message="Got colour wheel data") -> ()  [unwired: 1 in, 1 out]
              }
              frame "Set all config data" {
                n102 = Variant To Data(error in=w340, type=w336, Variant=w339) -> (data=w337:T3, error out=w338:errorcluster)
              }
              frame "Set all config data" {
              }
            }
            n103 = call "Update API.vi"("Config"=w186, "Error In"=w185) -> ("Error Out"=w184:errorcluster)  [unwired: 9 in]
          }
          event Value Change {
            n104 = event-data() -> ("NewVal"=w349:T2)  [unwired: 1 in]
            n105 = case shown="\"Spectrum Setup Complete\"" w349 {
              tunnel: [w352 w354 w356 w360 w364 w368 w370 w373 w376 w378 w380 w382 w384 w386 w388] -> w351
              tunnel: w350 -> [w353 w355 w357 w361 w365 w369 w370 w374 w377 w379 w381 w383 w385 w387 w388]
              tunnel: w348 -> [_ _ _ w358 w362 w367 _ w371 w375 _ _ _ _ _ _]
              frame "Start" {
                n106 = call "Start API.vi"("Error In"=w353) -> ("Error Out"=w352:errorcluster)  [unwired: 10 in]
              }
              frame "Initialise Devices" {
                n107 = call "Initialise Devices API.vi"("Error In"=w355) -> ("Error Out"=w354:errorcluster)  [unwired: 10 in]
              }
              frame "Stop" {
                n108 = call "Stop API.vi"("Error In"=w357) -> ("Error Out"=w356:errorcluster)  [unwired: 10 in]
              }
              frame "Set DAQ data" {
                n109 = Unbundle By Name(w358) -> ("DAQ"=w359:T4)
                n110 = call "Set DAQ config API.vi"("DAQ config"=w359, "Error In"=w361) -> ("Error Out"=w360:errorcluster)  [unwired: 9 in]
              }
              frame "Set Scope data" {
                n111 = Unbundle By Name(w362) -> ("Scope"=w363:T17)
                n112 = call "Set scope config API.vi"("Scope"=w363, "Error In"=w365) -> ("Error Out"=w364:errorcluster)  [unwired: 9 in]
              }
              frame "Set Monochromator data" {
                n113 = Unbundle By Name(w367) -> ("Monochromator"=w366:T7)
                n114 = call "Set monochromator data API.vi"("Monochromator"=w366, "Error In"=w369) -> ("Error Out"=w368:errorcluster)  [unwired: 9 in]
              }
              frame "Spectrum Setup Complete" {
              }
              frame "Set colour wheel data" {
                n115 = Unbundle By Name(w371) -> ("Colour wheel"=w372:T29)
                n116 = call "Set colour wheel data API.vi"("Colour wheel"=w372, "Error In"=w374) -> ("Error Out"=w373:errorcluster)  [unwired: 9 in]
              }
              frame "Set all config data" {
                n117 = call "Set all config data API.vi"("Error In"=w377, "Config"=w375) -> ("Error Out"=w376:errorcluster)  [unwired: 8 in, 1 out]
              }
              frame "Acquire test data" {
                n118 = call "Acquire DAQ and scope data API.vi"("Error In"=w379) -> ("Error Out"=w378:errorcluster)  [unwired: 10 in]
              }
              frame "Accumulate test data" {
                n119 = call "Accumulate test data API.vi"("Error In"=w381) -> ("Error Out"=w380:errorcluster)  [unwired: 10 in]
              }
              frame "Average test data" {
                n120 = call "Average test data API.vi"("Error In"=w383) -> ("Error Out"=w382:errorcluster)  [unwired: 10 in]
              }
              frame "Finalise test data" {
                n121 = call "Finalise test data API.vi"("Error In"=w385) -> ("Error Out"=w384:errorcluster)  [unwired: 10 in]
              }
              frame "Process test data" {
                n122 = call "Process test data API.vi"("Error In"=w387) -> ("Error Out"=w386:errorcluster)  [unwired: 10 in]
              }
              frame "Set all config data" {
              }
            }
          }
          event User Event {
            n123 = event-data() -> ()  [unwired: 1 in, 5 out]
          }
        }
      }
      frame Error {
        n124 = local read "Standalone"() -> (w397:bool)
        n125 = case shown="False" w397 {
          tunnel: [w402 _] -> w398
          tunnel: w399 -> [w401 w407]
          frame False {
            n126 = case shown="Error" w401 {
              selector: w401 -> [w403 w405]
              tunnel: [w403 w406] -> w402
              frame No Error {
              }
              frame Error {
                n127 = call "Send Error API.vi"("Error Cluster"=w405) -> ("Error Out"=w404:errorcluster)  [unwired: 10 in]
                n128 = call "Log error API.vi"("Error In"=w404) -> ("Error Out"=w406:errorcluster)  [unwired: 10 in]
              }
            }
          }
          frame True {
            n129 = call <vilib>:"Simple Error Handler.vi"("error in (no error)"=w407) -> ()  [unwired: 4 in, 5 out]
          }
        }
      }
    }
    "Config out" <- w25
    "Current step" <- w20
  }
  "Error Out" <- w11
